vi "Handle Command.vi"(8 "error in":errorcluster, 10 "Change Laser Vrange in":refnum<class "Change Laser Vrange.lvclass">, 11 "Object In":refnum<class>) -> (0 "error out":errorcluster, 1 "Command Successful?":bool, 2 "Change Laser Vrange Out":refnum<class "Change Laser Vrange.lvclass">, 3 "Object Out":refnum<class>)   [LabVIEW 2018, in "ePAS Library.lvlib" / "Change Laser Vrange.lvclass"]
doc: "Abstract method for accomplishing the execution of a command directed to an instrument object on the wire."
uses:
  Change Laser Vrange.lvclass
  Instrument/ePAS.lvclass
  C:/Users/Labview/Documents/exscalabar_server/reusable/Instrument/Instrument.lvclass
  Change Laser Vrange.lvclass/Change Laser Vrange.ctl
  Instrument/ePAS.lvclass/ePAS.ctl
  reusable/Instrument/Instrument.lvclass/Instrument.ctl
  Instrument/Accessors/Read FPGA Session.vi
  reusable/Instrument/Read Log Session.vi
  <vilib>/Utility/error.llb/Error Cluster From Error Code.vi
  <vilib>/rvi/errors/niLvFpgaAdjustHostInterfaceError.vi
  <userlib>/_Session Fwk/Session - Root.lvclass
  <vilib>/rvi/interface/nirviReadWriteControl/nirviReadWriteControl.xnode
  FPGA/R FPGA Ref.ctl
  FPGA Bitfiles/FPGAServer.lvbitx
  FPGA/Session/Exscalabar FPGA.lvclass
  ePAS Library.lvlib
  reusable/Session APIs/Session Log/System Log.lvclass
  NiFpgaLv.dll
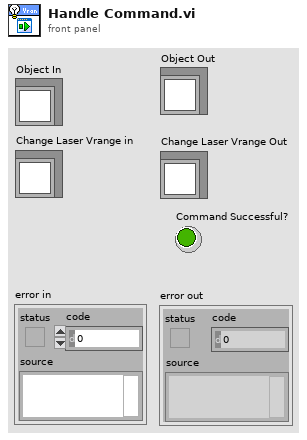
[diagram p1: front panel]
types:
  T1 = typedef "Session - Root.lvclass/Session Handle.ctl" = refnum<data-value>
  T2 = typedef "ePAS Library.lvlib/R FPGA Ref.ctl" = refnum<k20>
  T3 = cluster{"f0":fxp<+,32,0>, "Scale":fxp<+,32,0>, "Offset":i16, "Mod":enum8{"Sine", "Square"}}
  T4 = cluster{"f0":fxp<+,32,0>, "Scale":fxp<+,32,0>, "Offset":i16, "Mod":enum8{"Sine", "Square"}}[]
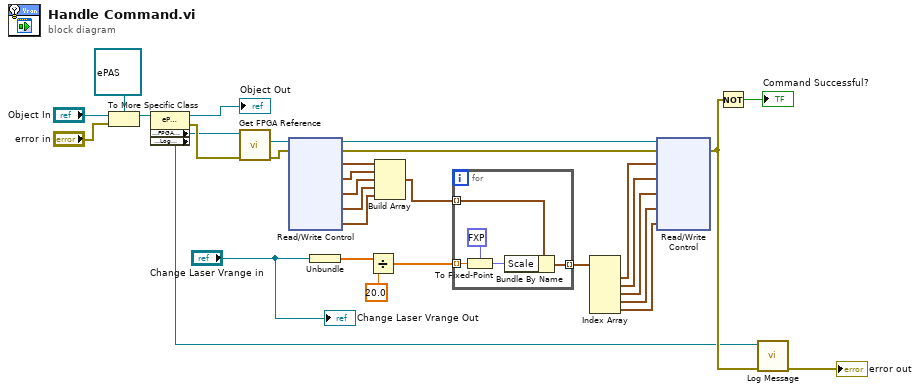
[diagram p0: block diagram]
diagram:
  n1 = To More Specific Class(target class=refnum<class "ePAS.lvclass"> refnum ("ePAS"), reference="Object In", error in="error in") -> (specific class reference=w5:refnum<class "ePAS.lvclass">)  [unwired: 1 out]
  n2 = property class="ePAS"(reference=w5) -> (reference out=→"Object Out":refnum<class "ePAS.lvclass">, error out=w4:errorcluster, "Accessors:FPGA Session"=w2:T1, "Accessors:Log Session"=w6:T1)  [unwired: 1 in]
  n3 = call "Get FPGA Reference.vi"("error in"=w4, "Session In"=w2) -> ("error out"=w13:errorcluster, "Ex FPGA Ref"=w29:T2)  [unwired: 7 in, 1 out]
  n4 = xnode "Read/Write Control"("FPGA VI Reference In"=w29, "error in"=w13) -> ("FPGA VI Reference Out"=w22:T2, "error out"=w21:errorcluster, "Cell 1"=w28:T3, "Cell 2"=w27:T3, "Cell 3"=w26:T3, "Cell 4"=w25:T3, "Cell 5"=w24:T3)
  n5 = Unbundle("Change Laser Vrange in") -> (w8:dbl[])
  n6 = Divide(x=w8, y=20.0) -> (x/y=w11:dbl[])
  n7 = Build Array(w28, w27, w26, w25, w24) -> (w23:T4)
  n8 = for {
    tunnel: w23 -> [w36] mode=indexing
    tunnel: w11 -> [w35] mode=indexing
    tunnel: [w32] -> w20 mode=indexing
    n9 = To Fixed-Point(fixed-point type=fxp<+,32,0> 0.0 ("f0"), number=w35) -> (fixed-point=w33:fxp<+,32,0>)
    n10 = Bundle By Name(cluster=w36, "Scale"=w33) -> (w32:T3)
  }
  n11 = Index Array(array=w20) -> (element #1=w19:T3, element #2=w18:T3, element #3=w17:T3, element #4=w16:T3, element #5=w15:T3)  [unwired: 5 in]
  n12 = xnode "Read/Write Control"("FPGA VI Reference In"=w22, "error in"=w21, "Cell 1"=w19, "Cell 2"=w18, "Cell 3"=w17, "Cell 4"=w16, "Cell 5"=w15) -> ("error out"=w7:errorcluster)  [unwired: 1 out]
  n13 = Not(x=w7) -> (.not. x?=→"Command Successful?":bool)
  n14 = call "Log Message.vi"("error in"=w7, "session in"=w6) -> ("error out"=→"error out":errorcluster)  [unwired: 8 in, 1 out]
  "Change Laser Vrange Out" <- "Change Laser Vrange in"
